vi "Write.vi"(0 "reference in":refnum<class "ConfigJSON.lvclass">, 5 "Data":variant, 7 "Name":string, 11 "error in (no error)":errorcluster) -> (4 "reference out":refnum<class "ConfigJSON.lvclass">, 6 "Data dub":variant, 8 "Name dub":string, 15 "error out":errorcluster)   [LabVIEW 2019, in "ConfigJSON.lvclass"]
uses:
  ConfigJSON.lvclass
  ConfigJSON.lvclass/ConfigJSON.ctl
  <vilib>/addons/_JKI.lib/Serialization/JSON/JKI JSON Serialization.lvlib
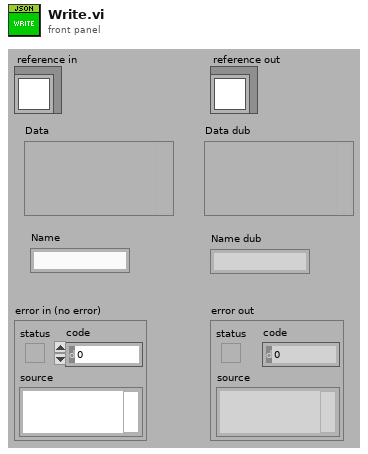
[diagram p1: front panel]
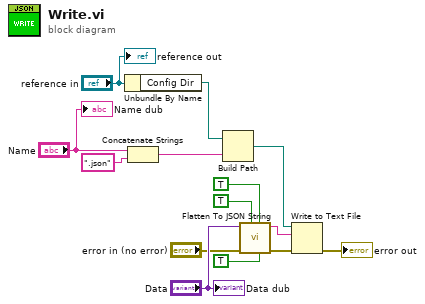
[diagram p0: block diagram]
diagram:
  n1 = Unbundle By Name("reference in") -> ("Config Dir"=w12:path)
  n2 = Concatenate Strings("Name", ".json" ("string")) -> (w10:string)
  n3 = Build Path(base path=w12, name or relative path=w10) -> (appended path=w9:path)
  n4 = call <vilib>:"Flatten To JSON String.vi"("Enums As String (F)"=TRUE, "Numeric Extensions (F)"=TRUE, "Multiline (T)"=TRUE, "error in (no error)"="error in (no error)", "Variant"="Data") -> ("error out"=w5:errorcluster, "JSON String"=w8:string)  [unwired: 5 in]
  n5 = Write to Text File(file (use dialog)=w9, text=w8, error in=w5) -> (error out=→"error out":errorcluster)  [unwired: 1 in, 2 out]
  "reference out" <- "reference in"
  "Name dub" <- "Name"
  "Data dub" <- "Data"
